vi "testCustomAssertionFailureMessage.vi"() -> ()   [LabVIEW 2017, in "AssertionTest.lvlib" / "AssertNotCount.lvlib"]
uses:
  AssertNotCount.lvlib
  Assertion/Assertion.lvlib
panel:
  out "error out":errorcluster
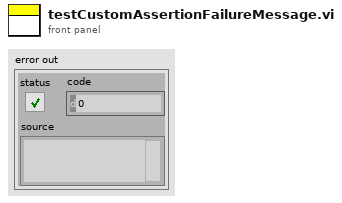
[diagram p1: front panel]
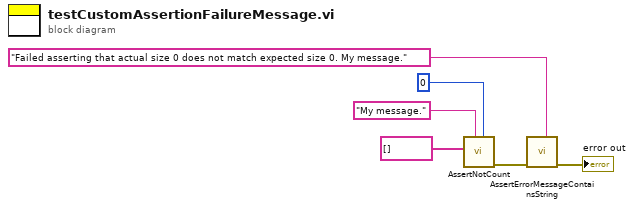
[diagram p0: block diagram]
diagram:
  n1 = call "AssertNotCount.vi"("Expected"=0, "Message (\"\")"="My message." ("Message (\"\")"), "Haystack"=string[] []) -> ("error out"=w6:errorcluster)  [unwired: 8 in]
  n2 = call "AssertErrorMessageContainsString.vi"("Expected"="Failed asserting that actual size 0 does not match expected size 0. My message." ("y"), "error in (no error)"=w6) -> ("error out"=→"error out":errorcluster)  [unwired: 9 in]
